vi "FPGA_CounterConvertModeToEdgeType.vi"(10 "Mode":T1, 11 "Edges":T3={"UpRisingEdge"=TRUE, "UpFallingEdge"=TRUE, "DownRisingEdge"=TRUE, "DownFallingEdge"=TRUE}) -> (3 "EdgeType":T2={"Master Mode"=enum."Edge Detection", "UpChannel"=enum."Disabled", "DownChannel"=enum."Disabled", "High/Up"=FALSE})   [LabVIEW 2017]
uses:
  <vilib>/Rock Robotics/SystemInterfaces/Counter/FPGA_CounterCtrEdgeDetectionType.ctl
  <vilib>/Rock Robotics/SystemInterfaces/Counter/FPGA_CounterEventCtrMode.ctl
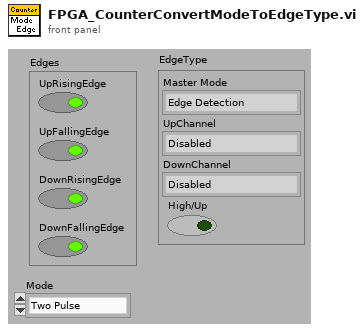
[diagram p1: front panel]
types:
  T1 = typedef "FPGA_CounterEventCtrMode.ctl" = enum8{"Two Pulse", "Semiperiod", "Pulse Length", "External Direction"}
  T2 = typedef "FPGA_CounterCtrEdgeDetectionType.ctl" = cluster{"Master Mode":enum16{"Edge Detection", "Semi Period Mode", "Pulse Length Mode", "External Direction"}, "UpChannel":enum16{"Rising Edge", "Falling Edge", "Raising & Falling Edge", "Disabled"}, "DownChannel":enum16{"Rising Edge", "Falling Edge", "Raising & Falling Edge", "Disabled"}, "High/Up":bool}
  T3 = cluster{"UpRisingEdge":bool, "UpFallingEdge":bool, "DownRisingEdge":bool, "DownFallingEdge":bool}
  T4 = enum16{"Edge Detection", "Semi Period Mode", "Pulse Length Mode", "External Direction"}
  T5 = enum16{"Rising Edge", "Falling Edge", "Raising & Falling Edge", "Disabled"}
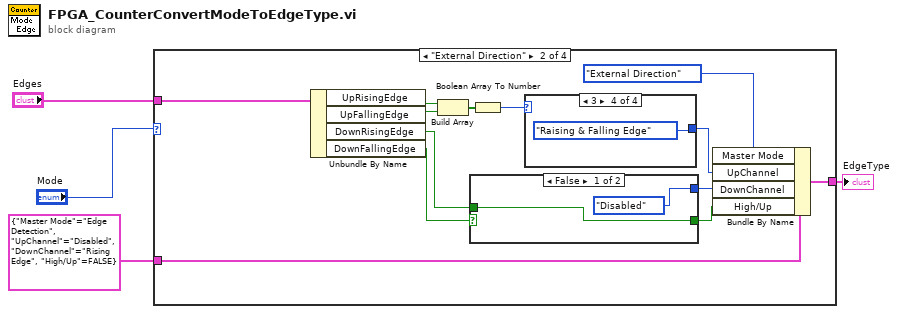
[diagram p0: block diagram]
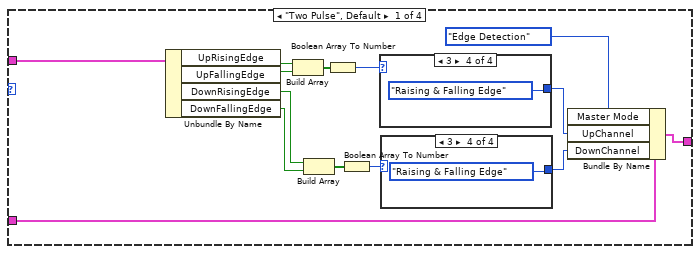
[diagram p2: hidden frame]
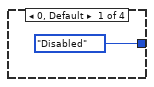
[diagram p3: hidden frame]
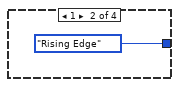
[diagram p4: hidden frame]
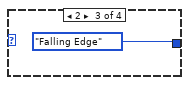
[diagram p5: hidden frame]
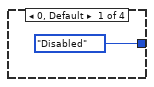
[diagram p6: hidden frame]
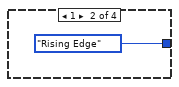
[diagram p7: hidden frame]
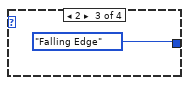
[diagram p8: hidden frame]
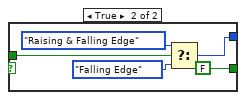
[diagram p9: hidden frame]
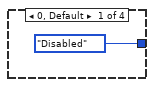
[diagram p10: hidden frame]
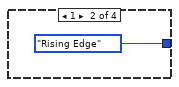
[diagram p11: hidden frame]
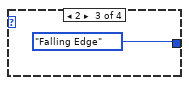
[diagram p12: hidden frame]
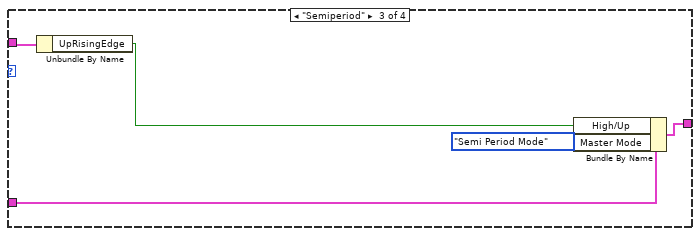
[diagram p13: hidden frame]
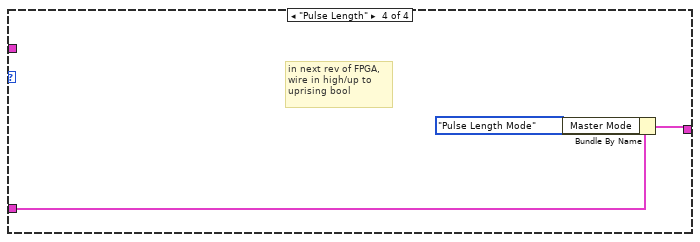
[diagram p14: hidden frame]
diagram:
  n1 = case shown="\"External Direction\"" "Mode" {
    tunnel: T2 {"Master Mode"=enum."Edge Detection", "UpChannel"=enum."Disabled", "DownChannel"=enum."Rising Edge", "High/Up"=FALSE} ("Edge") -> [w18 w39 w55 w56]
    tunnel: [w17 w38 w54 w57] -> w3
    tunnel: "Edges" -> [w16 w37 w52 _]
    frame "Two Pulse", Default {
      n2 = Unbundle By Name(w16) -> ("UpRisingEdge"=w15:bool, "UpFallingEdge"=w14:bool, "DownRisingEdge"=w6:bool, "DownFallingEdge"=w11:bool)
      n3 = Build Array(w15, w14) -> (w13:bool[])
      n4 = Build Array(w6, w11) -> (w12:bool[])
      n5 = Boolean Array To Number(Boolean array=w13) -> (number=w10:u32)
      n6 = Boolean Array To Number(Boolean array=w12) -> (number=w8:u32)
      n7 = case shown="3" w10 {
        tunnel: [T5."Disabled" ("UpChannel") T5."Rising Edge" ("UpChannel") T5."Falling Edge" ("UpChannel") T5."Raising & Falling Edge" ("UpChannel")] -> w9
        frame 0, Default {
        }
        frame 1 {
        }
        frame 2 {
        }
        frame 3 {
        }
      }
      n8 = case shown="3" w8 {
        tunnel: [T5."Disabled" ("UpChannel") T5."Rising Edge" ("UpChannel") T5."Falling Edge" ("UpChannel") T5."Raising & Falling Edge" ("UpChannel")] -> w7
        frame 0, Default {
        }
        frame 1 {
        }
        frame 2 {
        }
        frame 3 {
        }
      }
      n9 = Bundle By Name(cluster=w18, "Master Mode"=T4."Edge Detection", "UpChannel"=w9, "DownChannel"=w7) -> (w17:T2)
    }
    frame "External Direction" {
      n10 = Unbundle By Name(w37) -> ("UpRisingEdge"=w36:bool, "UpFallingEdge"=w35:bool, "DownRisingEdge"=w29:bool, "DownFallingEdge"=w30:bool)
      n11 = Build Array(w36, w35) -> (w34:bool[])
      n12 = case shown="False" w30 {
        tunnel: w29 -> [w41 w44]
        tunnel: [w41 FALSE ("DownRisingEdge")] -> w28
        tunnel: [T5."Disabled" ("UpChannel") w45] -> w27
        frame False {
        }
        frame True {
          n13 = Select(t=T5."Raising & Falling Edge" ("UpChannel"), s=w44, f=T5."Falling Edge" ("UpChannel")) -> (s? t:f=w45:T5)
        }
      }
      n14 = Boolean Array To Number(Boolean array=w34) -> (number=w33:u32)
      n15 = case shown="3" w33 {
        tunnel: [T5."Disabled" ("UpChannel") T5."Rising Edge" ("UpChannel") T5."Falling Edge" ("UpChannel") T5."Raising & Falling Edge" ("UpChannel")] -> w32
        frame 0, Default {
        }
        frame 1 {
        }
        frame 2 {
        }
        frame 3 {
        }
      }
      n16 = Bundle By Name(cluster=w39, "Master Mode"=T4."External Direction", "UpChannel"=w32, "DownChannel"=w27, "High/Up"=w28) -> (w38:T2)
    }
    frame "Semiperiod" {
      n17 = Unbundle By Name(w52) -> ("UpRisingEdge"=w51:bool)
      n18 = Bundle By Name(cluster=w55, "High/Up"=w51, "Master Mode"=T4."Semi Period Mode") -> (w54:T2)
    }
    frame "Pulse Length" {
      # "in next rev of FPGA,\nwire in high/up to \nuprising bool"
      n19 = Bundle By Name(cluster=w56, "Master Mode"=T4."Pulse Length Mode") -> (w57:T2)
    }
  }
  "EdgeType" <- w3
